vi "normalize graph.vi"(1 "Primary Graph":cluster{cluster{"x":dbl, "x":dbl}[]}[](graph) caption="cpsgraph") -> (0 "Normalized Primary Graph":cluster{cluster{"x":dbl, "x":dbl}[]}[](graph) caption="cpsgraph")   [LabVIEW 2017]
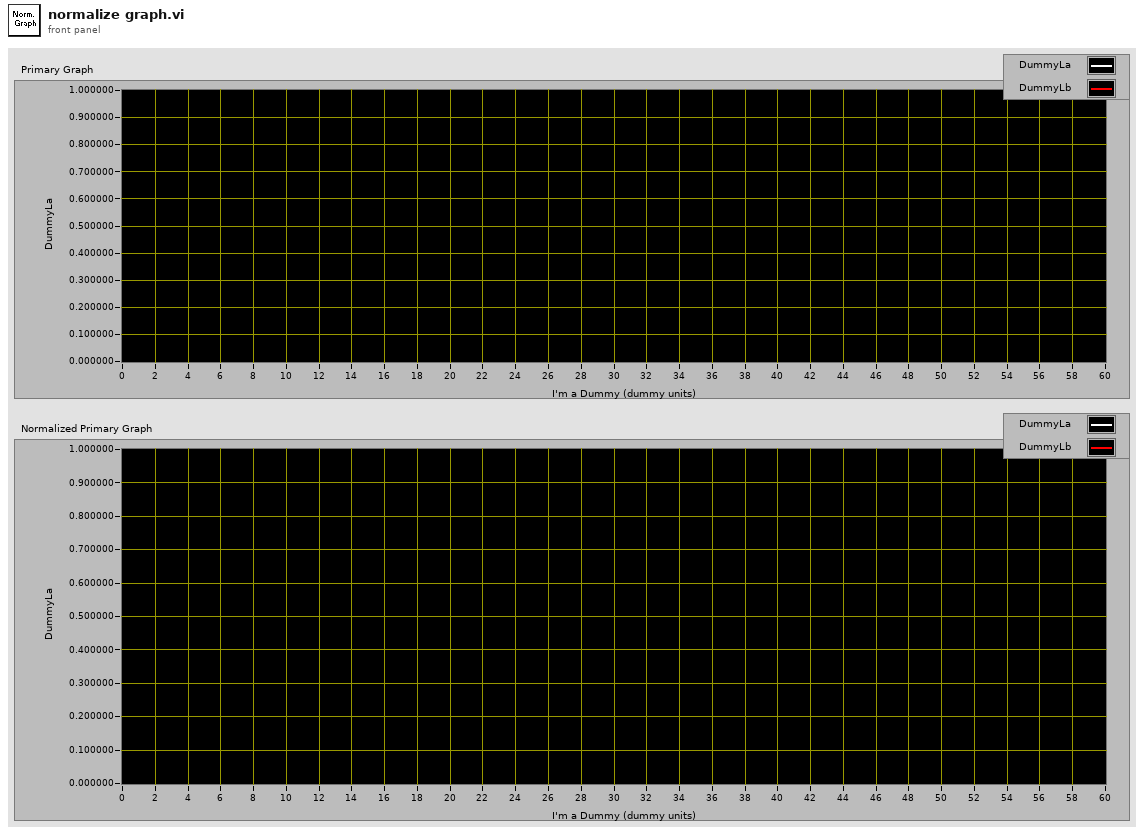
[diagram p1: front panel]
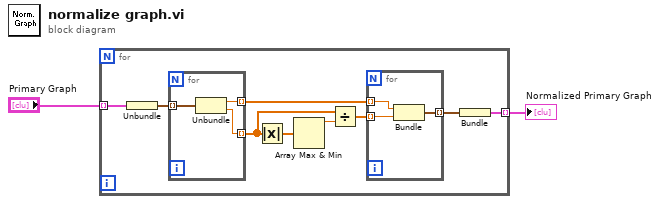
[diagram p0: block diagram]
diagram:
  n1 = for {
    tunnel: "Primary Graph" -> [w11] mode=indexing
    tunnel: [w3] -> w2 mode=indexing
    n2 = Unbundle(w11) -> (w10:cluster{"x":dbl, "x":dbl}[])
    n3 = for {
      tunnel: w10 -> [w17] mode=indexing
      tunnel: [w16] -> w6 mode=indexing
      tunnel: [w15] -> w8 mode=indexing
      n4 = Unbundle(w17) -> ("x"=w16:dbl, "x"=w15:dbl)
    }
    n5 = Absolute Value(x=w8) -> (abs(x)=w9:dbl[])
    n6 = Array Max & Min(array=w9) -> (max value=w7:dbl)  [unwired: 3 out]
    n7 = Divide(x=w8, y=w7) -> (x/y=w5:dbl[])
    n8 = for {
      tunnel: w6 -> [w14] mode=indexing
      tunnel: w5 -> [w13] mode=indexing
      tunnel: [w12] -> w4 mode=indexing
      n9 = Bundle("x"=w14, w13) -> (w12:cluster{"x":dbl, dbl})  [unwired: 1 in]
    }
    n10 = Bundle(w4) -> (w3:cluster{cluster{"x":dbl, dbl}[]})  [unwired: 1 in]
  }
  "Normalized Primary Graph" <- w2
